vi "DeCoF exec.vi"(0 "Conncection ID in":T1, 5 "command":string, 7 "argument 1":string, 9 "argument 2":string, 11 "error in":errorcluster) -> (4 "Conncection ID out":T1, 8 "answer string":string, 15 "error out":errorcluster)   [LabVIEW 2013]
uses:
  subVIs/DeCoF connection.ctl
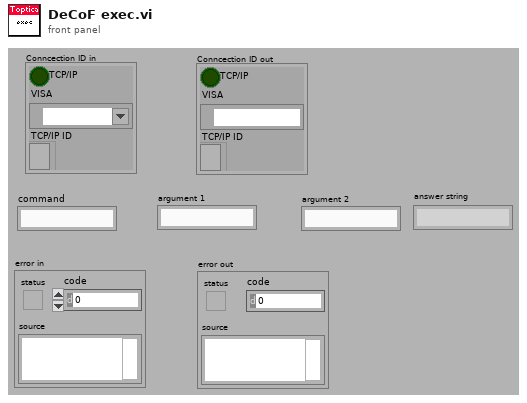
[diagram p1: front panel]
types:
  T1 = typedef "DeCoF connection.ctl" = cluster{"TCP/IP":bool, "VISA":refnum<visa-resource-name>, "TCP/IP ID":refnum<k5>}
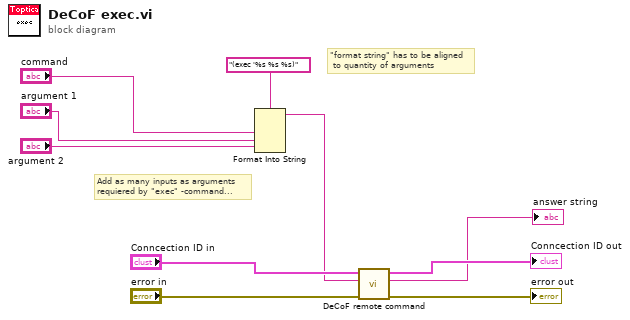
[diagram p0: block diagram]
diagram:
  # "\"format string\" has to be aligned\n to quantity of arguments"
  # "Add as many inputs as arguments \nrequiered by \"exec\" -command..."
  n1 = Format Into String(format string="(exec '%s %s %s)", "command", "argument 1", "argument 2") -> (resulting string=w6:string)  [unwired: 2 in, 1 out]
  n2 = call "DeCoF remote command.vi"("error in (no error)"="error in", "command"=w6, "Conncection ID in"="Conncection ID in") -> ("error out"=→"error out":errorcluster, "answer string"=→"answer string":string, "Conncection ID out"=→"Conncection ID out":T1)  [unwired: 2 in, 2 out]
